vi "Start.vi"() -> (2 "ªì©l°ïÅ|ª©":bool[][](array[boolean]))   [LabVIEW 2013]
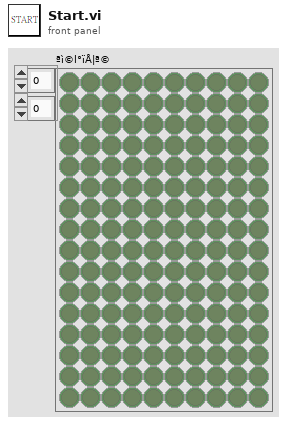
[diagram p1: front panel]
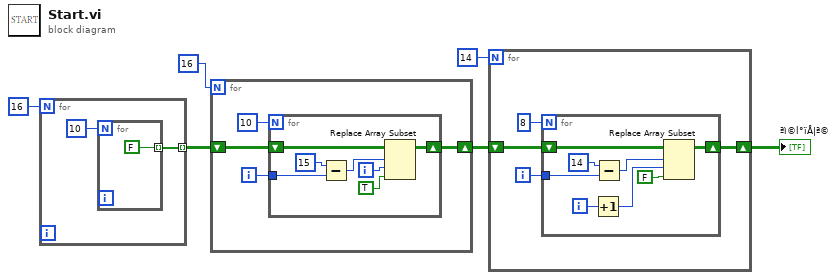
[diagram p0: block diagram]
diagram:
  n1 = for {
    N: 16 -> [_]
    tunnel: [w7] -> w2 mode=indexing
    n2 = for {
      N: 10 -> [_]
      tunnel: [FALSE] -> w7 mode=indexing
    }
  }
  n3 = for {
    N: 16 -> [_]
    shift-right: [w11] -> w5
    shift-left: w2 -> [w12]
    i -> [w10]
    n4 = for {
      N: 10 -> [_]
      shift-right: [w18] -> w11
      shift-left: w12 -> [w19]
      tunnel: w10 -> [w14]
      i -> [w17]
      n5 = Subtract(x=15, y=w14) -> (x-y=w15:i32)
      n6 = Replace Array Subset(array=w19, new element=TRUE, index (row)=w15, index (col)=w17) -> (w18:bool[][])
    }
  }
  n7 = for {
    N: 14 -> [_]
    shift-right: [w22] -> w1
    shift-left: w5 -> [w24]
    i -> [w21]
    n8 = for {
      N: 8 -> [_]
      shift-right: [w31] -> w22
      shift-left: w24 -> [w32]
      tunnel: w21 -> [w30]
      i -> [w27]
      n9 = Increment(x=w27) -> (x+1=w26:i32)
      n10 = Subtract(x=14, y=w30) -> (x-y=w29:i32)
      n11 = Replace Array Subset(array=w32, new element=FALSE ("new element/subarray"), index (row)=w29, index (col)=w26) -> (w31:bool[][])
    }
  }
  "ªì©l°ïÅ|ª©" <- w1
